vi "START EDIT USER.vi"(10 "USER/ITEM DATA TRANSFER":T2(array[cluster]), 11 "REFERENCES":T3) -> (2 "User Image":T4, 3 "USER INFO OUT":T1)   [LabVIEW 2019]
uses:
  <vilib>/vision/Image Controls.llb/IMAQ Image.ctl
  Controls/References Cluster.ctl
  <vilib>/userDefined/High Color/IMAQdx.ctl
  Controls/Custom Calendar/Custom Calendar.xctl
  <vilib>/Utility/miscctls.llb/LVStringsAndValuesArrayTypeDef_U16.ctl
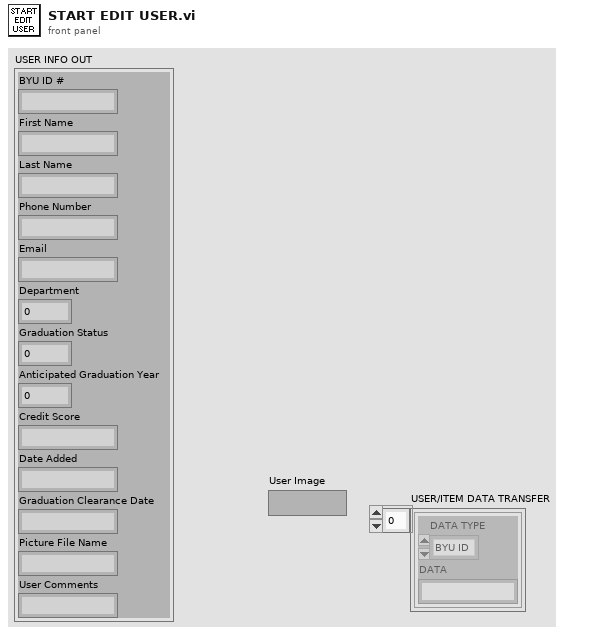
[diagram p1: front panel]
types:
  T1 = cluster{"BYU ID #":string, "First Name":string, "Last Name":string, "Phone Number":string, "Email":string, "Department":u16, "Graduation Status":u16, "Anticipated Graduation Year":u16, "Credit Score":string, "Date Added":string, "Graduation Clearance Date":string, "Picture File Name":string, "User Comments":string}
  T2 = cluster{"DATA TYPE":enum16{"BYU ID", "ME#/IDENTIFIER", "BYU ICN"}, "DATA":string}[]
  T3 = typedef "References Cluster.ctl" = cluster{"MAIN PAGES":refnum<vi>, "ADD/EDIT ITEM REFERENCES":cluster{"Identifier":refnum<vi>, "BYU ICN #":refnum<vi>, "Item Description":refnum<vi>, "Comments":refnum<vi>, "Checked Out Date":refnum<vi>, "Due Date":refnum<vi>, "Check Out Location":refnum<vi>, "Reminder Count":refnum<vi>, "Most Recent Reminder Date":refnum<vi>, "BYU ID #":refnum<vi>, "Building/Room":refnum<vi>, "Location in Room":refnum<vi>, "Manual":refnum<vi>, "Manufacturer":refnum<vi>, "Model #":refnum<vi>, "Serial #":refnum<vi>, "Date Acquired":refnum<vi>, "ADD/EDIT ITEM LABEL":refnum<vi>, "ARCHIVE ITEM":refnum<vi>, "Archive Item Inputs":refnum<vi>, "Reminder Notes":refnum<vi>, "DUPLICATE ITEM":refnum<vi>}, "ADD/EDIT USER REFERENCES":cluster{"BYU ID # (##-###-####)":refnum<vi>, "First Name":refnum<vi>, "Last Name":refnum<vi>, "Phone Number (###-###-####)":refnum<vi>, "Email":refnum<vi>, "Department":refnum<vi>, "Graduation Status":refnum<vi>, "Anticipated Graduation Year":refnum<vi>, "Credit Score":refnum<vi>, "Date Added":refnum<vi>, "Graduation Clearance Date":refnum<vi>, "Picture File Name":refnum<vi>, "ADD/EDIT USER LABEL":refnum<vi>, "Department Map":refnum<vi>, "Status Map":refnum<vi>, "Anticipated Graduation Year Map":refnum<vi>, "User Agreement":refnum<vi>, "User Comments":refnum<vi>, "Camera":refnum<vi>}, "RETURN ITEM REFERENCES":cluster{"Item or Person:":refnum<vi>, "Search Return Results":refnum<vi>, "What are you searching for?":refnum<vi>}, "SEARCH DATABASE REFERENCES":cluster{"What to Search For:":refnum<vi>, "Where to Search":refnum<vi>, "Column to Search In":refnum<vi>, "Column to Sort By":refnum<vi>, "Search Database Results":refnum<vi>, "Inventory Column Selector":refnum<vi>, "User Column Selector":refnum<vi>, "Inventory Archive Column Selector":refnum<vi>, "User Archive Column Selector":refnum<vi>, "Sales Tracking Column Selector":refnum<vi>, "Checked In Archive Column Selector":refnum<vi>, "Restore User":refnum<vi>, "Date Range":refnum<vi>, "Dates Less Than":refnum<vi>, "Dates Greater Than":refnum<vi>, "Search Print Receipt":refnum<vi>, "Edit Sale Description":refnum<vi>}, "USER ITEMS REFERENCES":cluster{"USER'S INFORMATION":refnum<vi>, "User's Checked Out Items":refnum<vi>, "User Info Comments":refnum<vi>, "SEE USER INFO COMMENTS":refnum<vi>}, "EDIT ITEMS REFERENCES":cluster{"New Check Out Location":refnum<vi>, "Items to Edit":refnum<vi>, "Edit Items Due Date":refnum<vi>, "New Reminder Notes":refnum<vi>, "New Item Description":refnum<vi>}, "CHECK OUT ITEMS REFERENCES":cluster{"Enter Item:":refnum<vi>, "Check Out Items Due Date":refnum<vi>, "Check Out Location":refnum<vi>, "Items to be Checked Out":refnum<vi>, "Possible Items":refnum<vi>, "Altered Item Description":refnum<vi>}, "TRANSFER ITEMS REFERENCES":cluster{"Search Parameter":refnum<vi>, "What to Match":refnum<vi>, "Matching Individuals":refnum<vi>, "Items to be Transferred":refnum<vi>}, "SETTINGS REFERENCES":cluster{"PSC Database Settings":refnum<vi>, "PSC Sales Item Spreadsheet":refnum<vi>}, "PSC SALES REFERENCES":cluster{"BYU ID CARD #":refnum<vi>, "Sale Description":refnum<vi>, "Scan or Enter Item Name":refnum<vi>, "Items to be Sold":refnum<vi>, "Grand Total":refnum<vi>, "Item List":refnum<vi>}}
  T4 = typedef "IMAQ Image.ctl" = refnum<image>
  T5 = typedef "LVStringsAndValuesArrayTypeDef_U16.ctl" = cluster{"String":string, "Value":u16}[]
  T6 = enum8{"Enabled", "Disabled", "Disabled and Grayed Out"}
  T7 = enum32{"IDLE", "ADD/EDIT USER", "ADD/EDIT ITEM", "RETURN ITEMS", "SEARCH DATABASE", "USER ITEMS", "CHECK OUT ITEMS", "EDIT ITEMS", "TRANSFER ITEMS", "PSC SALES", "ATRIUM", "INVENTORY TRACKING", "SETTINGS"}
  T8 = typedef "LVDateTimeRec.ctl" = cluster{"fractional second":dbl, "second":i32, "minute":i32, "hour":i32, "day of month":i32, "month":i32, "year":i32, "day of week":i32, "day of year":i32, "DST":i32}
  T9 = cluster{"BYU ID # (##-###-####)":refnum<vi>, "First Name":refnum<vi>, "Last Name":refnum<vi>, "Phone Number (###-###-####)":refnum<vi>, "Email":refnum<vi>, "Department":refnum<vi>, "Graduation Status":refnum<vi>, "Anticipated Graduation Year":refnum<vi>, "Credit Score":refnum<vi>, "Date Added":refnum<vi>, "Graduation Clearance Date":refnum<vi>, "Picture File Name":refnum<vi>, "ADD/EDIT USER LABEL":refnum<vi>, "Department Map":refnum<vi>, "Status Map":refnum<vi>, "Anticipated Graduation Year Map":refnum<vi>, "User Agreement":refnum<vi>, "User Comments":refnum<vi>, "Camera":refnum<vi>}
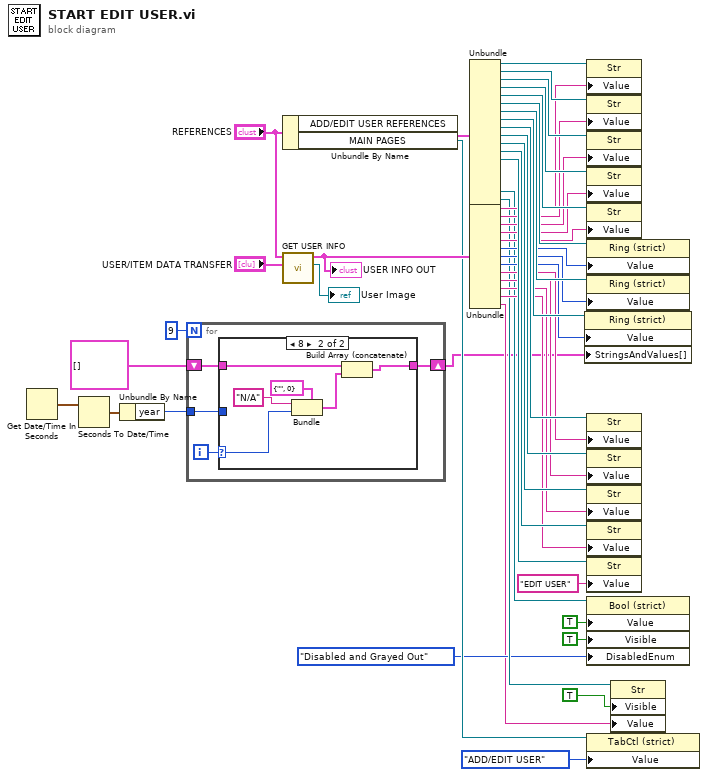
[diagram p0: block diagram]
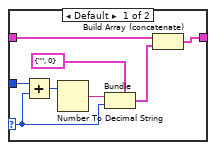
[diagram p2: hidden frame]
diagram:
  n1 = Get Date/Time In Seconds() -> (seconds since 1Jan1904=w2:timestamp)
  n2 = Seconds To Date/Time(time stamp (now)=w2) -> (date time rec=w4:T8)  [unwired: 1 in]
  n3 = Unbundle By Name(w4) -> ("year"=w3:i32)
  n4 = for {
    N: 9 -> [_]
    shift-right: [w47] -> w1
    shift-left: T5 [] ("Strings And Values []") -> [w49]
    tunnel: w3 -> [w48]
    i -> [w50]
    n5 = case shown="8" w50 {
      selector: w50 -> [w54 w59]
      tunnel: w49 -> [w53 w64]
      tunnel: w48 -> [w58 _]
      tunnel: [w51 w63] -> w47
      frame Default {
        n6 = Add(x=w58, y=w54) -> (x+y=w57:i32)
        n7 = Number To Decimal String(number=w57) -> (decimal integer string=w55:string)  [unwired: 1 in]
        n8 = Bundle(cluster=cluster{"String":string, "Value":u16} {"String"="", "Value"=0}, "String"=w55, "Value"=w54) -> (w52:cluster{"String":string, "Value":u16})
        n9 = Build Array (concatenate)(w53, w52) -> (w51:T5)
      }
      frame 8 {
        n10 = Bundle(cluster=cluster{"String":string, "Value":u16} {"String"="", "Value"=0}, "String"="N/A", "Value"=w59) -> (w60:cluster{"String":string, "Value":u16})
        n11 = Build Array (concatenate)(w64, w60) -> (w63:T5)
      }
    }
  }
  n12 = Unbundle By Name("REFERENCES") -> ("ADD/EDIT USER REFERENCES"=w20:T9, "MAIN PAGES"=w16:refnum<vi>)
  n13 = call "GET USER INFO.vi"("USER/ITEM DATA TRANSFER IN"="USER/ITEM DATA TRANSFER", "REFERENCES"="REFERENCES") -> ("User Image"=→"User Image":T4, "USER INFO OUT"=w17:T1)  [unwired: 8 in]
  "USER INFO OUT" <- w17
  n14 = Unbundle(w20) -> ("BYU ID # (##-###-####)"=w46:refnum<vi>, "First Name"=w45:refnum<vi>, "Last Name"=w44:refnum<vi>, "Phone Number (###-###-####)"=w43:refnum<vi>, "Email"=w42:refnum<vi>, "Department"=w41:refnum<vi>, "Graduation Status"=w40:refnum<vi>, "Anticipated Graduation Year"=w39:refnum<vi>, "Credit Score"=w38:refnum<vi>, "Date Added"=w37:refnum<vi>, "Graduation Clearance Date"=w36:refnum<vi>, "Picture File Name"=w35:refnum<vi>, "ADD/EDIT USER LABEL"=w34:refnum<vi>, "User Agreement"=w14:refnum<vi>, "User Comments"=w11:refnum<vi>)  [unwired: 4 out]
  n15 = Unbundle(w17) -> ("BYU ID #"=w32:string, "First Name"=w31:string, "Last Name"=w30:string, "Phone Number"=w29:string, "Email"=w28:string, "Department"=w27:u16, "Graduation Status"=w26:u16, "Anticipated Graduation Year"=w25:u16, "Credit Score"=w24:string, "Date Added"=w23:string, "Graduation Clearance Date"=w22:string, "Picture File Name"=w21:string, "User Comments"=w8:string)
  n16 = property class="Ring (strict)"(reference=w39, "Value"=w25, "StringsAndValues[]"=w1) -> ()  [unwired: 1 in, 2 out]
  n17 = property class="Str"(reference=w46, "Value"=w32) -> ()  [unwired: 1 in, 2 out]
  n18 = property class="Str"(reference=w45, "Value"=w31) -> ()  [unwired: 1 in, 2 out]
  n19 = property class="Str"(reference=w44, "Value"=w30) -> ()  [unwired: 1 in, 2 out]
  n20 = property class="Str"(reference=w43, "Value"=w29) -> ()  [unwired: 1 in, 2 out]
  n21 = property class="Str"(reference=w42, "Value"=w28) -> ()  [unwired: 1 in, 2 out]
  n22 = property class="Ring (strict)"(reference=w41, "Value"=w27) -> ()  [unwired: 1 in, 2 out]
  n23 = property class="Ring (strict)"(reference=w40, "Value"=w26) -> ()  [unwired: 1 in, 2 out]
  n24 = property class="Str"(reference=w38, "Value"=w24) -> ()  [unwired: 1 in, 2 out]
  n25 = property class="Str"(reference=w37, "Value"=w23) -> ()  [unwired: 1 in, 2 out]
  n26 = property class="Str"(reference=w36, "Value"=w22) -> ()  [unwired: 1 in, 2 out]
  n27 = property class="Str"(reference=w35, "Value"=w21) -> ()  [unwired: 1 in, 2 out]
  n28 = property class="Str"(reference=w34, "Value"="EDIT USER") -> ()  [unwired: 1 in, 2 out]
  n29 = property class="Bool (strict)"(reference=w14, "Value"=TRUE, "Visible"=TRUE, "DisabledEnum"=T6."Disabled and Grayed Out" ("Disabled")) -> ()  [unwired: 1 in, 2 out]
  n30 = property class="TabCtl (strict)"(reference=w16, "Value"=T7."ADD/EDIT USER") -> ()  [unwired: 1 in, 2 out]
  n31 = property class="Str"(reference=w11, "Visible"=TRUE, "Value"=w8) -> ()  [unwired: 1 in, 2 out]
